vi "SQL_StoreCountersMonitor.vi"(8 "Counters Monitor Array":T1(array[cluster]), 9 "SubAssembly":string, 10 "LineName":string, 11 "ConnectionDSN":string) -> ()   [LabVIEW 2017]
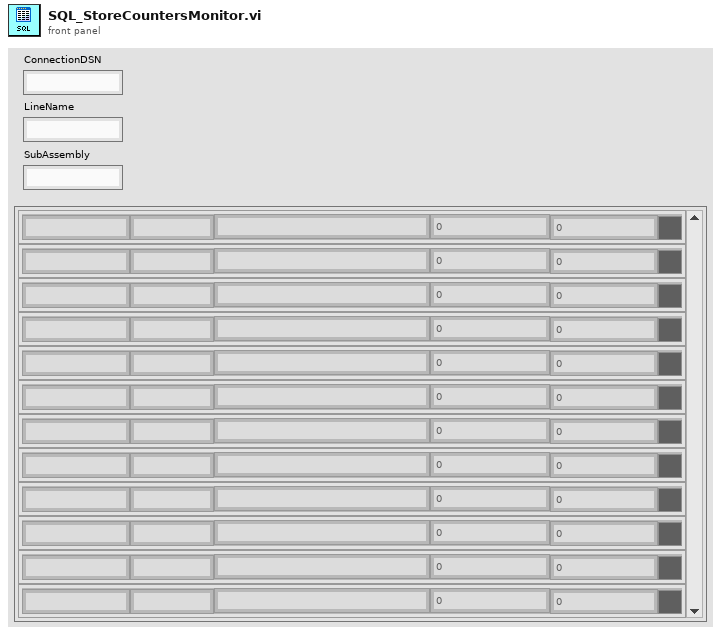
[diagram p1: front panel]
types:
  T1 = cluster{"MachineName":string, "ComponentName":string, "StoppageAlarmCounter":i32, "CurrentCount":i32, "StatusColorBox":u32, "ToolCribPartNumber":string}[]
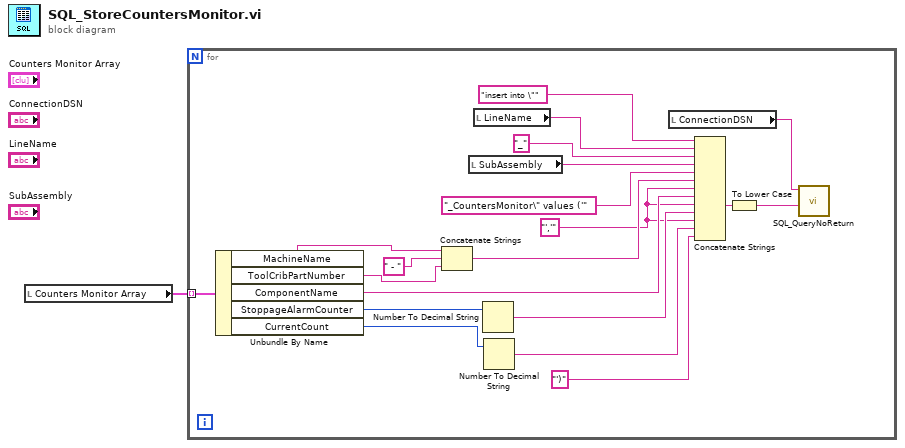
[diagram p0: block diagram]
diagram:
  n1 = local read "Counters Monitor Array"() -> (w1:T1)
  n2 = for {
    tunnel: w1 -> [w21] mode=indexing
    w10 = "','"
    n3 = Unbundle By Name(w21) -> ("MachineName"=w17:string, "ToolCribPartNumber"=w15:string, "ComponentName"=w12:string, "StoppageAlarmCounter"=w20:i32, "CurrentCount"=w19:i32)
    n4 = Concatenate Strings(w17, " - ", w15) -> (w13:string)
    n5 = local read "SubAssembly"() -> (w5:string)
    n6 = local read "LineName"() -> (w3:string)
    n7 = Number To Decimal String(number=w20) -> (decimal integer string=w11:string)  [unwired: 1 in]
    n8 = Number To Decimal String(number=w19) -> (decimal integer string=w9:string)  [unwired: 1 in]
    n9 = local read "ConnectionDSN"() -> (w6:string)
    n10 = Concatenate Strings("insert into \"", w3, "_", w5, "_CountersMonitor\" values ('", w13, w10, w12, w10, w11, w10, w9, "')") -> (w18:string)
    n11 = To Lower Case(string=w18) -> (all lower case string=w7:string)
    n12 = call "SQL_QueryNoReturn.vi"("SQL query"=w7, "ConnectionDSN"=w6) -> ()  [unwired: 10 in]
  }
